vi "Part 1.vi"(11 "Input":string) -> (3 "Output":i64)   [LabVIEW 2021]
uses:
  <userlib>/_OpenG.lib/string/string.llb/Convert EOLs (String)__ogtk.vi
  Module/Module.lvclass
panel:
  out "Low Pulses":i64
  out "High Pulses":i64
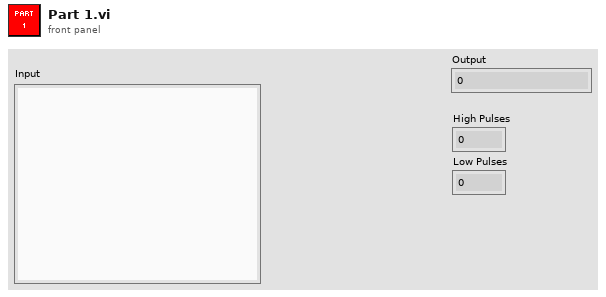
[diagram p1: front panel]
types:
  T1 = cluster{"From":string, "To":string, "Pulse":bool}
  T2 = cluster{"From":string, "To":string, "Pulse":bool}[]
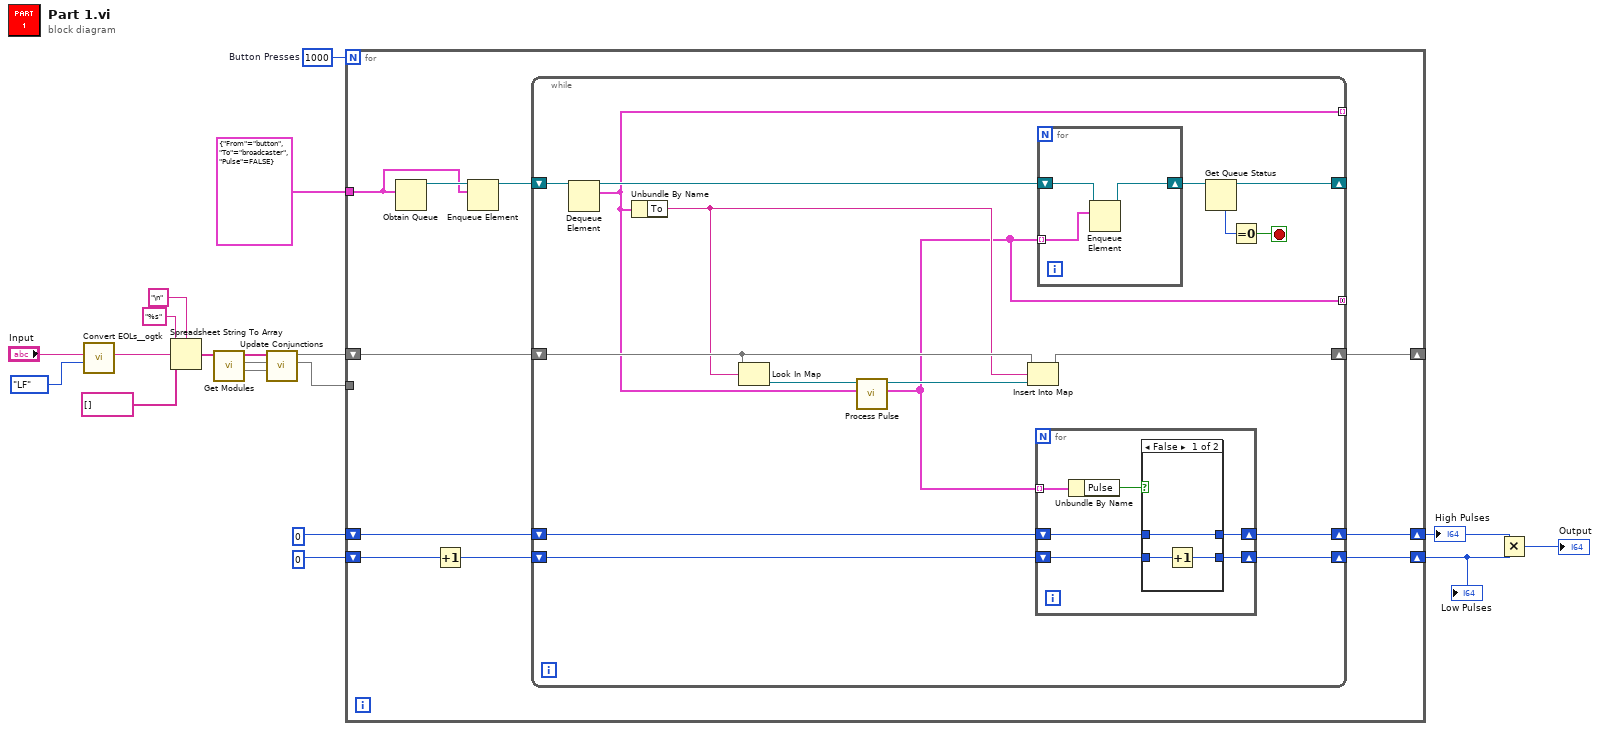
[diagram p0: block diagram]
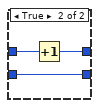
[diagram p2: hidden frame]
diagram:
  w9 = 1000  # Button Presses
  n1 = call-poly <userlib>:"Convert EOLs__ogtk.vi"("Convert to:"=enum16{"CR", "LF", "CRLF"}."LF", "String in"="Input") -> ("String out"=w15:string)  [unwired: 9 in]
  n2 = Spreadsheet String To Array(delimiter (Tab)="\n", format string="%s", spreadsheet string=w15, array type (2D Dbl)=string[] []) -> (array=w13:string[])
  n3 = call "Get Modules.vi"("Module list in"=w13) -> ("Destination Map"=w10:map{string, string[]}, "Module Map"=w11:map{string, refnum<class "Module.lvclass">}, "Conjunctions out"=w12:string[])  [unwired: 8 in]
  n4 = call "Update Conjunctions.vi"("Destination Map in"=w10, "Module Map in"=w11, "Conjunctions in"=w12) -> ("Destination Map out"=w7:map{string, string[]}, "Module Map out"=w8:map{string, refnum<class "Module.lvclass">})  [unwired: 7 in]
  n5 = for {
    N: w9 -> [_]
    shift-right: [w28] -> _
    shift-left: w8 -> [w29]
    tunnel: w7 -> [_]
    tunnel: T1 {"From"="button", "To"="broadcaster", "Pulse"=FALSE} -> [w21]
    shift-right: [w25] -> w2
    shift-left: i64 0 -> [w26]
    shift-right: [w23] -> w3
    shift-left: i64 0 -> [w24]
    n6 = Obtain Queue(element data type=w21) -> (queue out=w27:refnum<queue>)  [unwired: 4 in, 2 out]
    n7 = Increment(x=w24) -> (x+1=w20:i64)
    n8 = Enqueue Element(queue=w27, element=w21) -> (queue out=w22:refnum<queue>)  [unwired: 2 in, 2 out]
    n9 = while {
      shift-right: [w39] -> w28
      shift-left: w29 -> [w42]
      shift-right: [w45] -> _
      shift-left: w22 -> [w44]
      shift-right: [w35] -> w25
      shift-left: w26 -> [w36]
      shift-right: [w33] -> w23
      shift-left: w20 -> [w34]
      tunnel: [w32] -> _ mode=concatenating
      tunnel: [w31] -> _ mode=indexing
      stop <- w30 stop-if-true
      n10 = Dequeue Element(queue=w44) -> (queue out=w38:refnum<queue>, element=w31:T1)  [unwired: 2 in, 2 out]
      n11 = Unbundle By Name(w31) -> ("To"=w41:string)
      n12 = Look In Map(map=w42, key=w41) -> (value=w43:refnum<class "Module.lvclass">)  [unwired: 1 in, 1 out]
      n13 = call-dynamic "Process Pulse.vi"("Input"=w31, "Module in"=w43) -> ("Outputs"=w32:T2, "Module out"=w40:refnum<class "Module.lvclass">)  [unwired: 7 in, 1 out]
      n14 = Insert Into Map(map in=w42, key=w41, value=w40) -> (map out=w39:map{string, refnum<class "Module.lvclass">})  [unwired: 2 out]
      n15 = for {
        tunnel: w32 -> [w52] mode=indexing
        shift-right: [w49] -> w35
        shift-left: w36 -> [w50]
        shift-right: [w47] -> w33
        shift-left: w34 -> [w48]
        n16 = Unbundle By Name(w52) -> ("Pulse"=w51:bool)
        n17 = case shown="False" w51 {
          tunnel: w50 -> [w55 w58]
          tunnel: [w55 w57] -> w49
          tunnel: w48 -> [w54 w56]
          tunnel: [w53 w56] -> w47
          frame False {
            n18 = Increment(x=w54) -> (x+1=w53:i64)
          }
          frame True {
            n19 = Increment(x=w58) -> (x+1=w57:i64)
          }
        }
      }
      n20 = for {
        shift-right: [w59] -> w37
        shift-left: w38 -> [w61]
        tunnel: w32 -> [w60] mode=indexing
        n21 = Enqueue Element(queue=w61, element=w60) -> (queue out=w59:refnum<queue>)  [unwired: 2 in, 2 out]
      }
      n22 = Get Queue Status(queue=w37) -> (queue out=w45:refnum<queue>, # elements in queue=w46:i32)  [unwired: 2 in, 6 out]
      n23 = Equal To 0?(x=w46) -> (x = 0?=w30:bool)
    }
  }
  "High Pulses" <- w2
  "Low Pulses" <- w3
  n24 = Multiply(x=w2, y=w3) -> (x*y=→"Output":i64)
